vi "Configure.vi"(7 "Reset":bool, 8 "error in (no error)":errorcluster, 9 "baud rate (9600)":u32=9600, 10 "VISA resource name":refnum<visa-resource-name>="COM2", 11 "Serial Controller in":refnum<class "Serial Controller.lvclass">) -> (0 "error out":errorcluster, 3 "Serial Controller out":refnum<class "Serial Controller.lvclass">)   [LabVIEW 2012, in "Serial Controller.lvclass"]
uses:
  Serial Controller.lvclass
  <vilib>/Instr/_visa.llb/VISA Set IO Buffer Mask.ctl
  Serial Controller.lvclass/Serial Controller.ctl
  <vilib>/Instr/_visa.llb/VISA Configure Serial Port (Instr).vi
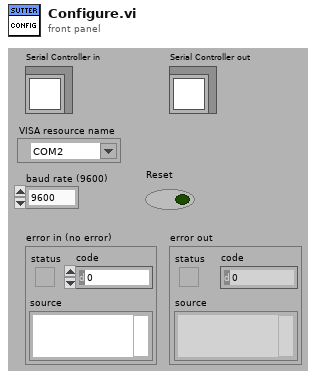
[diagram p1: front panel]
types:
  T1 = typedef "VISA Set IO Buffer Mask.ctl" = u16
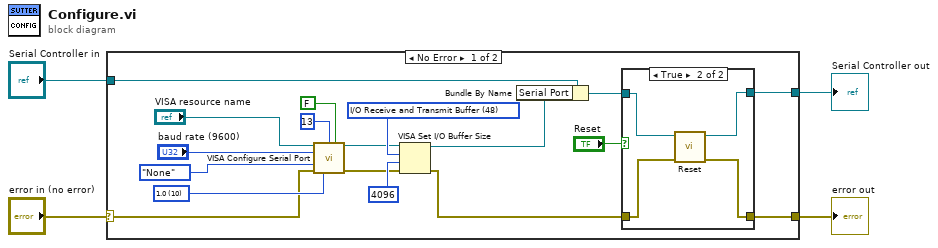
[diagram p0: block diagram]
diagram:
  n1 = case shown="No Error" "error in (no error)" {
    selector: "error in (no error)" -> [w16 w30]
    tunnel: [w6 w30] -> w3
    tunnel: [w7 w29] -> w1
    tunnel: "Serial Controller in" -> [w15 w29]
    frame No Error {
      w14 = T1 48 items=["I/O Receive Buffer"=16, "I/O Transmit Buffer"=32, "I/O Receive and Transmit Buffer"=48] ("Mask")
      w17 = u16 10 items=["1.0"=10, "1.5"=15, "2.0"=20] ("stop bits (10: 1 bit)")
      n2 = call-poly "VISA Configure Serial Port"("VISA resource name"="VISA resource name", "termination char\n(0xA = '\\n' = LF)"=u8 13 ("termination char\n(0xA = '\\n' = LF)"), "Enable Termination\nChar (T)"=FALSE ("Enable Termination\nChar (T)"), "baud rate (9600)"="baud rate (9600)", "parity (0:none)"=enum16{"None", "Odd", "Even", "Mark", "Space"}."None", "error in (no error)"=w16, "stop bits (10: 1 bit)"=w17) -> ("VISA resource name out"=w12:refnum<visa-resource-name>, "error out"=w11:errorcluster)  [unwired: 7 in]
      n3 = VISA Set I/O Buffer Size(VISA resource name=w12, mask (16)=w14, size (4096)=u32 4096, error in (no error)=w11) -> (VISA resource name out=w10:refnum<visa-resource-name>, error out=w5:errorcluster)
      n4 = Bundle By Name(cluster=w15, "Serial Port"=w10) -> (w8:refnum<class "Serial Controller.lvclass">)
      n5 = case shown="True" "Reset" {
        tunnel: w8 -> [w24 w28]
        tunnel: [w24 w27] -> w7
        tunnel: [w23 w26] -> w6
        tunnel: w5 -> [w23 w25]
        frame False {
        }
        frame True {
          n6 = call-dynamic "Reset.vi"("error in (no error)"=w25, "Serial Controller in"=w28) -> ("error out"=w26:errorcluster, "Serial Controller out"=w27:refnum<class "Serial Controller.lvclass">)  [unwired: 8 in]
        }
      }
    }
    frame Error {
    }
  }
  "error out" <- w3
  "Serial Controller out" <- w1
